vi "myRIO_BRig_RT_comm_webdav_sendData_all.vi"(9 "Host Filename Prefix":string="Test", 10 "Host Password":string="sabalab", 11 "Host UserName":string="Test2") -> ()   [LabVIEW 2014]
panel:
  out "Connected To Host?":bool
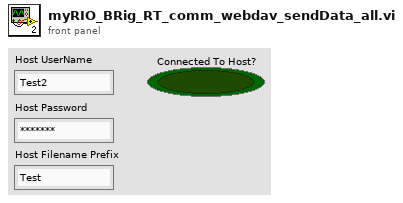
[diagram p1: front panel]
types:
  T1 = typedef "NI_WebDAV.lvlib/SessionHandle.ctl" = refnum<k1>
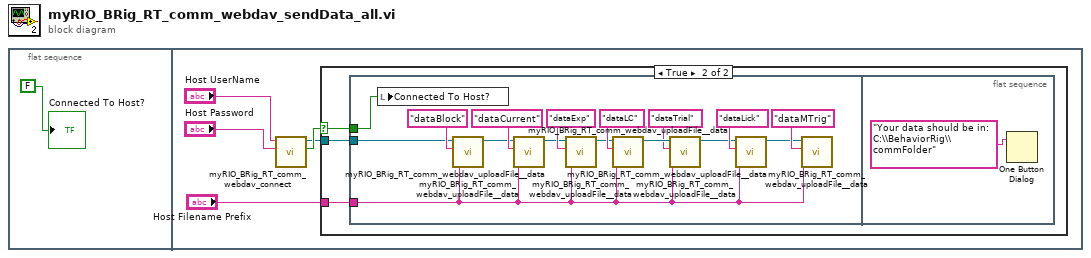
[diagram p0: block diagram]
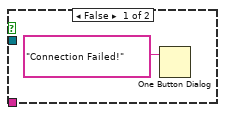
[diagram p2: hidden frame]
diagram:
  n1 = flat-sequence {
    frame #0 {
      "Connected To Host?" <- FALSE
    }
    frame #1 {
      n2 = call "myRIO_BRig_RT_comm_webdav_connect.vi"("input_password"="Host Password", "input_username"="Host UserName") -> ("output_Iconnected"=w4:bool, "output_hSession"=w3:T1)  [unwired: 7 in, 1 out]
      n3 = case shown="True" w4 {
        selector: w4 -> [_ w10]
        tunnel: w3 -> [_ w9]
        tunnel: "Host Filename Prefix" -> [_ w8]
        frame False {
          n4 = One Button Dialog(message="Connection Failed!") -> ()  [unwired: 1 in, 1 out]
        }
        frame True {
          n5 = flat-sequence {
            tunnel: w10 -> [w26]
            tunnel: w9 -> [w24]
            tunnel: w8 -> [w11]
            frame #0 {
              n6 = local write "Connected To Host?"(w26) -> ()
              n7 = call "myRIO_BRig_RT_comm_webdav_uploadFile__data.vi"("input_fileName_prefix"=w11, "input_fileName"="dataBlock" ("input_filename"), "input_hSession"=w24) -> ("output_hSession"=w22:T1)  [unwired: 8 in]
              n8 = call "myRIO_BRig_RT_comm_webdav_uploadFile__data.vi"("input_fileName_prefix"=w11, "input_fileName"="dataCurrent" ("input_filename"), "input_hSession"=w22) -> ("output_hSession"=w20:T1)  [unwired: 8 in]
              n9 = call "myRIO_BRig_RT_comm_webdav_uploadFile__data.vi"("input_fileName_prefix"=w11, "input_fileName"="dataExp" ("input_filename"), "input_hSession"=w20) -> ("output_hSession"=w18:T1)  [unwired: 8 in]
              n10 = call "myRIO_BRig_RT_comm_webdav_uploadFile__data.vi"("input_fileName_prefix"=w11, "input_fileName"="dataLC" ("input_filename"), "input_hSession"=w18) -> ("output_hSession"=w17:T1)  [unwired: 8 in]
              n11 = call "myRIO_BRig_RT_comm_webdav_uploadFile__data.vi"("input_fileName_prefix"=w11, "input_fileName"="dataTrial" ("input_filename"), "input_hSession"=w17) -> ("output_hSession"=w14:T1)  [unwired: 8 in]
              n12 = call "myRIO_BRig_RT_comm_webdav_uploadFile__data.vi"("input_fileName_prefix"=w11, "input_fileName"="dataLick" ("input_filename"), "input_hSession"=w14) -> ("output_hSession"=w12:T1)  [unwired: 8 in]
              n13 = call "myRIO_BRig_RT_comm_webdav_uploadFile__data.vi"("input_fileName_prefix"=w11, "input_fileName"="dataMTrig" ("input_filename"), "input_hSession"=w12) -> ()  [unwired: 8 in, 1 out]
            }
            frame #1 {
              n14 = One Button Dialog(message="Your data should be in: C:\\BehaviorRig\\commFolder") -> ()  [unwired: 1 in, 1 out]
            }
          }
        }
      }
    }
  }
